vi "start.vi"(8 "error in (no error)":errorcluster, 10 "Load Cell Excitation":dbl[unit] format="%.1f", 11 "ForceSensor in":refnum<class "ForceSensorCalculator.lvclass">) -> (0 "error out":errorcluster, 3 "ForceSensor out":refnum<class "ForceSensorCalculator.lvclass">)   [LabVIEW 2015, in "ForceSensorCalculator.lvlib" / "ForceSensorCalculator.lvclass"]
uses:
  <userlib>/Common/Devices/ForceSensorCalculator/ForceSensorCalculator/ForceSensorCalculator.lvclass
  <userlib>/Common/Devices/ForceSensorCalculator/ForceSensorCalculator/ForceSensorCalculator.lvclass/ForceSensorCalculator.ctl
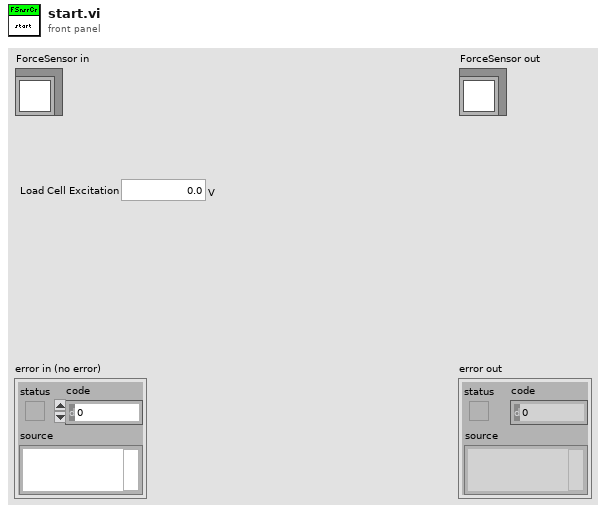
[diagram p1: front panel]
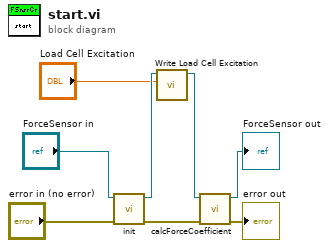
[diagram p0: block diagram]
diagram:
  n1 = call-dynamic "init.vi"("error in (no error)"="error in (no error)", "ForceSensor in"="ForceSensor in") -> ("error out"=w2:errorcluster, "ForceSensor out"=w4:refnum<class "ForceSensorCalculator.lvclass">)  [unwired: 8 in]
  n2 = call <userlib>:"Write Load Cell Excitation.vi"("Load Cell Excitation"="Load Cell Excitation", "ForceSensorCalculator in"=w4) -> ("ForceSensorCalculator out"=w3:refnum<class "ForceSensorCalculator.lvclass">)  [unwired: 9 in]
  n3 = call <userlib>:"calcForceCoefficient.vi"("error in (no error)"=w2, "ForceSensor in"=w3) -> ("error out"=→"error out":errorcluster, "ForceSensor out"=→"ForceSensor out":refnum<class "ForceSensorCalculator.lvclass">)  [unwired: 8 in]
